vi "getHallWaveformValues_minmaxrms_inAmps.vi"(0 "waveform in":waveform(dbl), 1 "Hall current sense scaling factor (mV/A)":dbl=40.0 format="%#_13g") -> (6 "DC (V)":dbl, 7 "minmax array (A)":dbl[](array[numeric]), 8 "max (A)":dbl=0.6054117299412742 format="%0.2f", 9 "min (A)":dbl=-0.6054117299412853 format="%0.2f", 10 "AC rms (A)":dbl)   [LabVIEW 2021]
panel:
  out "max (V)":dbl
  out "min (V)":dbl
  out "min - DC (V)":dbl
  out "max - DC (V)":dbl
  out "Waveform Graph":waveform(dbl)(graph)
  out "AC rms (V)":dbl
  out "total rms (V)":dbl
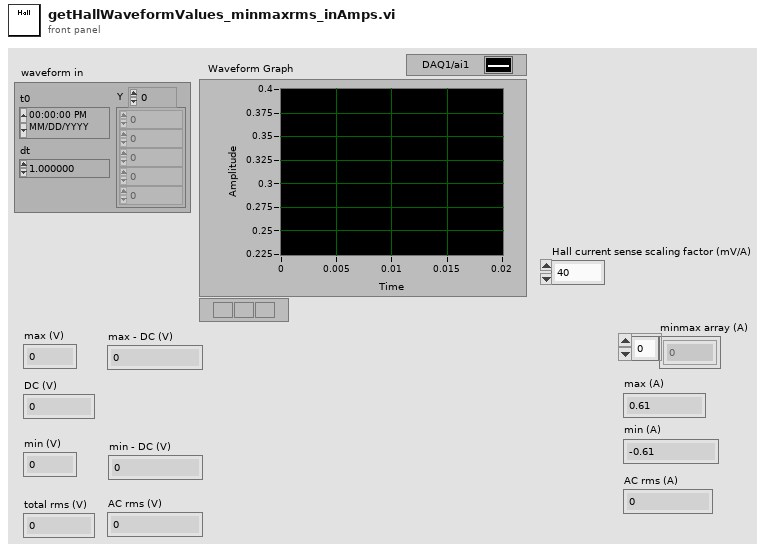
[diagram p1: front panel]
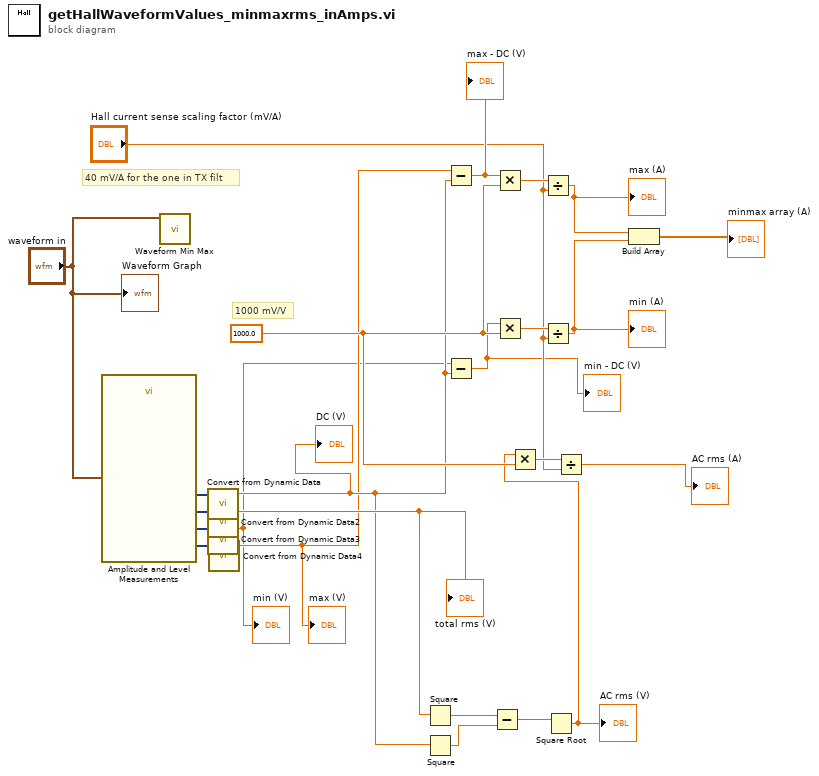
[diagram p0: block diagram]
diagram:
  w14 = 1000.0 ("y")
  # "1000 mV/V"
  # "40 mV/A for the one in TX filt"
  n1 = call "Amplitude and Level Measurements"("Signals"="waveform in") -> ("Mean (DC)"=w13:dynamicdata, "RMS"=w18:dynamicdata, "Negative Peak"=w5:dynamicdata, "Positive Peak"=w4:dynamicdata)  [unwired: 10 in, 1 out]
  n2 = call <vilib>:"Waveform Min Max.vi"("waveform in"="waveform in") -> ()  [unwired: 5 in, 6 out]
  n3 = call "Convert from Dynamic Data"("Dynamic Data Type"=w13) -> ("Scalar"=w8:dbl)  [unwired: 3 in]
  "DC (V)" <- w8
  n4 = call "Convert from Dynamic Data2"("Dynamic Data Type"=w18) -> ("Scalar"=w9:dbl)  [unwired: 3 in]
  "total rms (V)" <- w9
  n5 = call "Convert from Dynamic Data3"("Dynamic Data Type"=w5) -> ("Scalar"=w2:dbl)  [unwired: 3 in]
  "min (V)" <- w2
  n6 = call "Convert from Dynamic Data4"("Dynamic Data Type"=w4) -> ("Scalar"=w3:dbl)  [unwired: 3 in]
  "max (V)" <- w3
  n7 = Square(x=w9) -> (x^2=w12:dbl)
  n8 = Square(x=w8) -> (x^2=w11:dbl)
  n9 = Subtract(x=w3, y=w8) -> (x-y=w22:dbl)
  "max - DC (V)" <- w22
  n10 = Subtract(x=w2, y=w8) -> (x-y=w7:dbl)
  "min - DC (V)" <- w7
  n11 = Subtract(x=w12, y=w11) -> (x-y=w10:dbl)
  n12 = Multiply(x=w22, y=w14) -> (x*y=w24:dbl)
  n13 = Multiply(x=w7, y=w14) -> (x*y=w23:dbl)
  n14 = Divide(x=w24, y="Hall current sense scaling factor (mV/A)") -> (x/y=w21:dbl)
  "max (A)" <- w21
  n15 = Divide(x=w23, y="Hall current sense scaling factor (mV/A)") -> (x/y=w20:dbl)
  "min (A)" <- w20
  n16 = Square Root(x=w10) -> (sqrt(x)=w1:dbl)
  "AC rms (V)" <- w1
  n17 = Multiply(x=w1, y=w14) -> (x*y=w17:dbl)
  n18 = Divide(x=w17, y="Hall current sense scaling factor (mV/A)") -> (x/y=→"AC rms (A)":dbl)
  n19 = Build Array(w21, w20) -> (→"minmax array (A)":dbl[])
  "Waveform Graph" <- "waveform in"
